vi "Check Result Queue.vi"(8 "Error In":errorcluster, 10 "Averaging":T1 {"Traces" min=1 max=200 step=1}, 11 "Result Queue":refnum<queue>) -> (0 "Error Out":errorcluster, 2 "Ready":bool)   [LabVIEW 2017]
uses:
  Controls/Acquisition Result.ctl
  Averaging.ctl
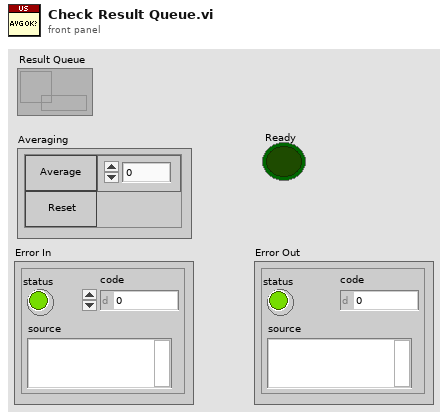
[diagram p1: front panel]
types:
  T1 = typedef "Averaging.ctl" = cluster{"On":bool, "Traces":i32, "Reset":bool}
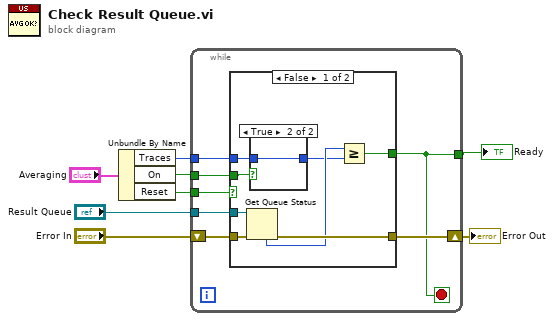
[diagram p0: block diagram]
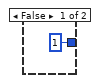
[diagram p2: hidden frame]
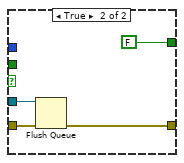
[diagram p3: hidden frame]
diagram:
  n1 = Unbundle By Name("Averaging") -> ("Traces"=w7:i32, "On"=w6:bool, "Reset"=w5:bool)
  n2 = while {
    tunnel: w7 -> [w14]
    tunnel: w5 -> [w12]
    tunnel: "Result Queue" -> [w11]
    shift-right: [w15] -> w8
    shift-left: "Error In" -> [w10]
    tunnel: w6 -> [w13]
    tunnel: [w9] -> w1
    stop <- w9 stop-if-true
    n3 = case shown="False" w12 {
      tunnel: [w23 w28] -> w15
      tunnel: w11 -> [w22 w27]
      tunnel: w14 -> [w18 _]
      tunnel: [w16 FALSE] -> w9
      tunnel: w13 -> [w19 _]
      tunnel: w10 -> [w20 w29]
      frame False {
        n4 = Get Queue Status(queue=w22, error in (no error)=w20) -> (error out=w23:errorcluster, # elements in queue=w21:i32)  [unwired: 1 in, 6 out]
        n5 = case shown="True" w19 {
          tunnel: [1 ("f") w25] -> w17
          tunnel: w18 -> [_ w25]
          frame False {
          }
          frame True {
          }
        }
        n6 = Greater Or Equal?(x=w21, y=w17) -> (x >= y?=w16:bool)
      }
      frame True {
        n7 = Flush Queue(queue=w27, error in (no error)=w29) -> (error out=w28:errorcluster)  [unwired: 2 out]
      }
    }
  }
  "Error Out" <- w8
  "Ready" <- w1
